vi "Configure.vi"(8 "error in (no error)":errorcluster, 11 "Common Measurements in":refnum<class "Common Measurements.lvclass">) -> (0 "error out":errorcluster, 3 "Common Measurements out":refnum<class "Common Measurements.lvclass">)   [LabVIEW 2015, in "Common Measurements.lvclass"]
uses:
  Common Measurements.lvclass
  Common Measurements Interface/Common Measurements Interface.lvclass
  Mag Lab Properties/Mag Lab Parameters.lvclass
  Mag Lab Measure Base/Mag Lab Measure Base.lvclass/Mag Lab Measure Base.ctl
  Mag Lab Root/Mag Lab Root.lvclass/Mag Lab Root.ctl
  Mag Lab Measure Controller/Mag Lab Measure Controller.lvclass/Mag Lab Measure Controller.ctl
  <vilib>/ActorFramework/Message Enqueuer/Message Enqueuer.lvclass/Message Enqueuer.ctl
  Mag Lab Root/Write Name.vi
  Mag Lab Root/Write Separate UI.vi
  <vilib>/ActorFramework/Message Enqueuer/Enqueue.vi
  <vilib>/ActorFramework/Message Priority Queue/Priority Enqueue.vi
  <vilib>/ActorFramework/Message Enqueuer/Message Enqueuer.lvclass
  Mag Lab Root Messages/Open Front Panel Msg/Open Front Panel Msg.lvclass
  Mag Lab Measure Controller/Mag Lab Measure Controller.lvclass
  Mag Lab Measure Base/Mag Lab Measure Base.lvclass
  Mag Lab Error Handler/Mag Lab Error Handler.lvclass
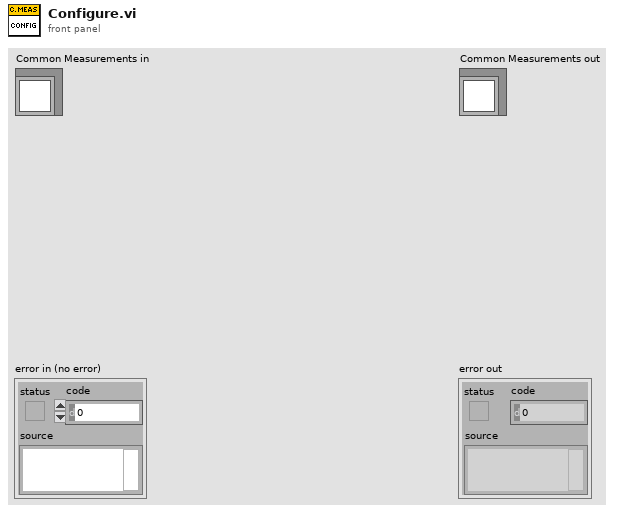
[diagram p1: front panel]
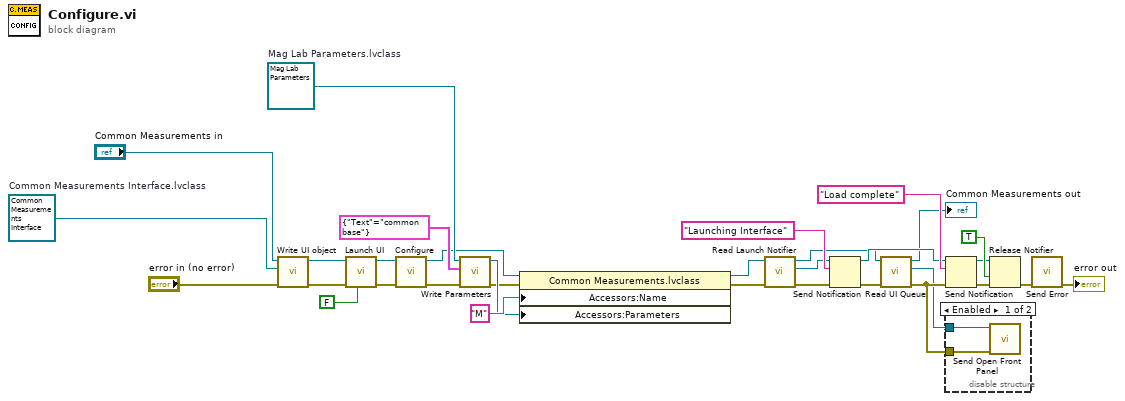
[diagram p0: block diagram]
diagram:
  w31 = refnum<class "Mag Lab Parameters.lvclass"> refnum  # Mag Lab Parameters.lvclass
  w32 = refnum<class "Common Measurements Interface.lvclass"> refnum  # Common Measurements Interface.lvclass
  n1 = call "Write UI object.vi"("error in (no error)"="error in (no error)", "Mag Lab Measure Interface.lvclass"=w32, "Mag Lab Measure Base in"="Common Measurements in") -> ("error out"=w11:errorcluster, "Mag Lab Measure Base out"=w14:refnum<class "Common Measurements.lvclass">)  [unwired: 7 in]
  n2 = call-dynamic "Launch UI.vi"("Auto-open"=FALSE, "error in (no error)"=w11, "Mag Lab Measure Base in"=w14) -> ("error out"=w15:errorcluster, "Mag Lab Measure Base out"=w16:refnum<class "Common Measurements.lvclass">)  [unwired: 7 in]
  n3 = call-parent "Configure.vi"("error in (no error)"=w15, "Mag Lab Measure Controller in"=w16) -> ("error out"=w29:errorcluster, "Mag Lab Measure Controller out"=w17:refnum<class "Common Measurements.lvclass">)  [unwired: 8 in]
  n4 = call-dynamic "Write Parameters.vi"("error in (no error)"=w29, "Parameters"=cluster{"Text":string} {"Text"="common base"}, "Mag Lab Parameters in"=w31) -> ("error out"=w18:errorcluster, "Mag Lab Parameters out"=w19:refnum<class "Mag Lab Parameters.lvclass">)  [unwired: 7 in]
  n5 = property class="Common Measurements.lvclass"(reference=w17, error in=w18, "Accessors:Name"="M" ("Name"), "Accessors:Parameters"=w19) -> (reference out=w10:refnum<class "Common Measurements.lvclass">, error out=w9:errorcluster)
  n6 = call "Read Launch Notifier.vi"("error in (no error)"=w9, "Mag Lab Measure Controller in"=w10) -> ("error out"=w21:errorcluster, "Launch Notifier"=w23:refnum<notifier>, "Mag Lab Measure Controller out"=w7:refnum<class "Common Measurements.lvclass">)  [unwired: 7 in]
  n7 = Send Notification(notification="Launching Interface" ("Message"), notifier=w23, error in (no error)=w21) -> (notifier out=w22:refnum<notifier>, error out=w8:errorcluster)
  n8 = call "Read UI Queue.vi"("error in (no error)"=w8, "Mag Lab Measure Base in"=w7) -> ("error out"=w5:errorcluster, "Actor Framework.lvlib:Message Enqueuer"=w2:refnum<class "Message Enqueuer.lvclass">, "Mag Lab Measure Base out"=→"Common Measurements out":refnum<class "Common Measurements.lvclass">)  [unwired: 7 in]
  n9 = Send Notification(notification="Load complete" ("Message"), notifier=w22, error in (no error)=w5) -> (notifier out=w25:refnum<notifier>, error out=w28:errorcluster)
  n10 = disable-structure shown="Enabled" {
    disable-tunnel: w5 -> [w34 _]
    disable-tunnel: w2 -> [w33 _]
    frame Enabled {
      n11 = call "Send Open Front Panel.vi"("error in (no error)"=w34, "Message Enqueuer"=w33) -> ()  [unwired: 8 in, 2 out]
    }
    frame Disabled {
    }
  }
  n12 = Release Notifier(notifier=w25, force destroy? (F)=TRUE ("Kill notifier"), error in (no error)=w28) -> (error out=w4:errorcluster)  [unwired: 2 out]
  n13 = call "Send Error.vi"("error in (no error)"=w4) -> ("error out"=→"error out":errorcluster)  [unwired: 9 in, 1 out]
